vi "Query IO.vi"(8 "error in":errorcluster, 11 "SL_SC in":refnum<class "SL_SC.lvclass">) -> (0 "error out":errorcluster, 1 "Port Array":u8[](array[numeric]), 2 "Boolean Array":bool[](array[boolean]), 3 "SL_SC out":refnum<class "SL_SC.lvclass">)   [LabVIEW 2019, in "SL_SC.lvlib" / "SL_SC.lvclass"]
doc: "This method must be overridden by the child class.\n\nThis should read the status at the output of the device and return a weform capture of the named signal states."
uses:
  Library/SL_SC.lvclass
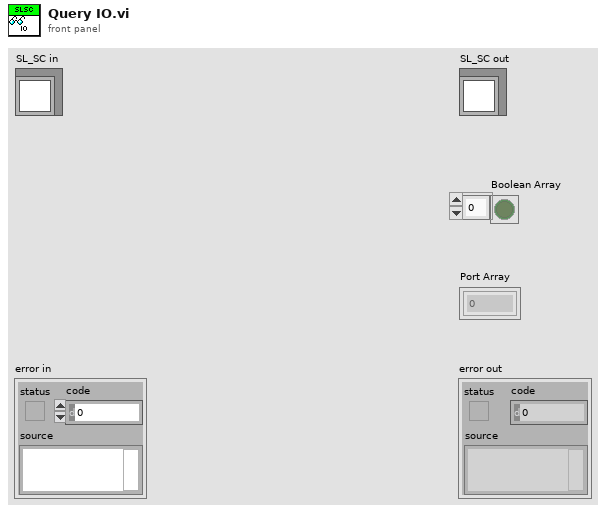
[diagram p1: front panel]
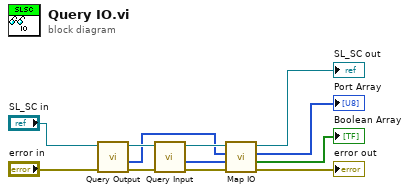
[diagram p0: block diagram]
diagram:
  n1 = call "Query Output.vi"("error in"="error in", "SL_SC in"="SL_SC in") -> ("error out"=w5:errorcluster, "Output"=w1:u8[], "SL_SC out"=w6:refnum<class "SL_SC.lvclass">)  [unwired: 7 in]
  n2 = call "Query Input.vi"("error in"=w5, "SL_SC in"=w6) -> ("error out"=w3:errorcluster, "Input"=w2:u8[], "SL_SC out"=w4:refnum<class "SL_SC.lvclass">)  [unwired: 7 in]
  n3 = call "Map IO.vi"("error in"=w3, "Input"=w2, "Output"=w1, "SL_SC in"=w4) -> ("error out"=→"error out":errorcluster, "Boolean Array"=→"Boolean Array":bool[], "Port Array"=→"Port Array":u8[], "SL_SC out"=→"SL_SC out":refnum<class "SL_SC.lvclass">)  [unwired: 4 in]
